vi "Create.vi"(8 "error in (no error)":errorcluster, 10 "UI Refs":T1) -> (0 "error out":errorcluster, 3 "Editor out":refnum<class "Editor.lvclass">, 4 "Event Reg":refnum<event-registration>)   [LabVIEW 2020, in "VolatusGUIEditor.lvlib" / "Editor.lvclass"]
uses:
  Editor.lvclass
  Editor.lvclass/Editor.ctl
  Control Bind Data.ctl
  VolatusGUIControls/VolatusGUIControls.lvlib
  Events.ctl
  UI Refs.ctl
  VolatusGUIEditor.lvlib
  Update Preview Data.ctl
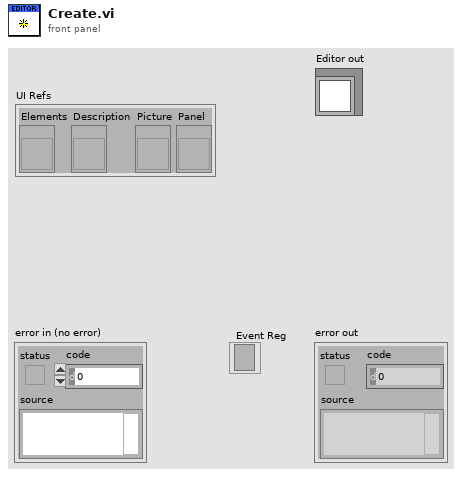
[diagram p1: front panel]
types:
  T1 = typedef "VolatusGUIEditor.lvlib/UI Refs.ctl" = cluster{"Elements":refnum<vi>, "Description":refnum<vi>, "Picture":refnum<vi>, "Panel":refnum<vi>}
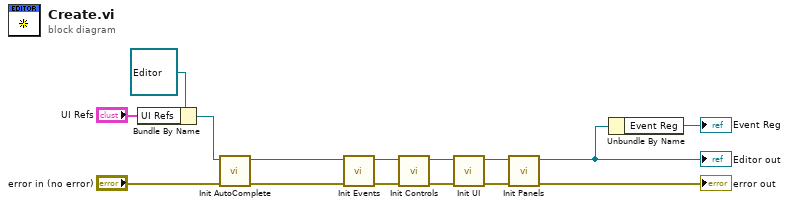
[diagram p0: block diagram]
diagram:
  n1 = Bundle By Name(cluster=refnum<class "Editor.lvclass"> refnum ("Editor in"), "UI Refs"="UI Refs") -> (w2:refnum<class "Editor.lvclass">)
  n2 = call "Init AutoComplete.vi"("error in (no error)"="error in (no error)", "Editor in"=w2) -> ("error out"=w3:errorcluster, "Editor out"=w1:refnum<class "Editor.lvclass">)  [unwired: 8 in]
  n3 = call "Init Events.vi"("error in (no error)"=w3, "Editor in"=w1) -> ("error out"=w14:errorcluster, "Editor out"=w7:refnum<class "Editor.lvclass">)  [unwired: 8 in]
  n4 = call "Init Controls.vi"("error in (no error)"=w14, "Editor in"=w7) -> ("error out"=w8:errorcluster, "Editor out"=w5:refnum<class "Editor.lvclass">)  [unwired: 8 in]
  n5 = call "Init UI.vi"("error in (no error)"=w8, "Editor in"=w5) -> ("error out"=w6:errorcluster, "Editor out"=w4:refnum<class "Editor.lvclass">)  [unwired: 8 in]
  n6 = call "Init Panels.vi"("error in (no error)"=w6, "Editor in"=w4) -> ("error out"=→"error out":errorcluster, "Editor out"=w11:refnum<class "Editor.lvclass">)  [unwired: 8 in]
  "Editor out" <- w11
  n7 = Unbundle By Name(w11) -> ("Event Reg"=→"Event Reg":refnum<event-registration>)
